vi "纳清DO电极校准.vi"() -> ()   [LabVIEW 2016, in "斯坦道多参数.lvlib"]
uses:
  <vilib>/Utility/miscctls.llb/LVPointTypeDef.ctl
  <vilib>/Utility/miscctls.llb/LVPositionTypeDef.ctl
  <vilib>/Analysis/NI_AALBase.lvlib
panel:
  out "盐度":sgl format="%#.2f"
  out "大气压力":sgl format="%#.2f"
  out "饱和值":sgl format="%#.2f"
  out "当前探头类别":string
  out "报警信息":string
  out "温度校准参数":sgl format="%#.2f"
  out "通讯状态":string
  out "第二点校准值":dbl
  out "第一点校准值":dbl
  in  "校准停止":bool
  in  "校准启动":bool
  in  "校准模式":enum16{"两点校准", "单点校准"}(ring)=enum."单点校准"
  out "最小值":sgl format="%#.2f"
  out "最大值":sgl format="%#.2f"
  out "波形图表":sgl(graph) caption="历史曲线"
  out "mean":dbl caption="均值" format="%#.2f"
  out "standard deviation":dbl caption="标准差" format="%#.2f"
  out "变异系数":dbl format="%#.6f"
  out "测量值":sgl format="%#.2f"
  out "提示":string
  out "原始光强数值":sgl caption="信号值" format="%#.6f"
  out "温度":dbl format="%#.2f"
  # "DO电极设定"
  # "℃"
  # "mg/L"
  # "%"
  # "nA"
  # "kPa"
  # "ppt"
  # "请选择校准模式:"
  # "℃"
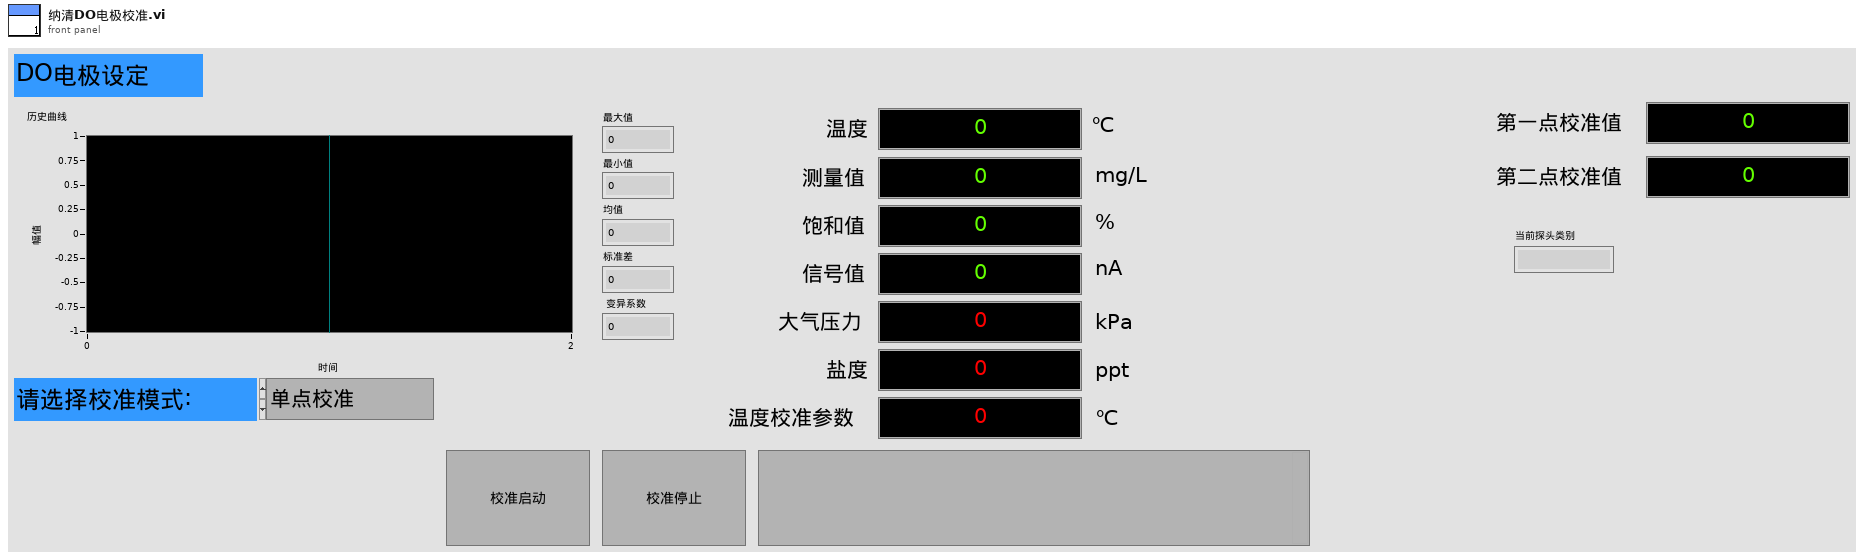
[diagram p1: front panel]
types:
  T1 = typedef "LVPointTypeDef.ctl" = cluster{"Horizontal":i16, "Vertical":i16}
  T2 = typedef "斯坦道多参数.lvlib/校准步骤.ctl" = enum16{"待机", "放置第一点标液", "第一点校准启动", "第一点校准写入", "第一点校准失败", "放置第二点标液", "第二点校准启动", "第二点校准写入", "第二点校准失败", "放置第三点标液", "第三点校准启动", "第三点校准写入", "第三点校准失败", "校准结果写入", "校准结束"}
  T3 = cluster{"报警码":u16, "溶解氧数值（mg/L）":sgl, "溶解氧数据（%）":sgl, "温度数据":sgl, "溶解氧原始信号 nA":sgl, "大气压力":sgl, "盐度":sgl, "0X0009_NC":string, "产品名称":string, "序列号":string, "硬件版本":string, "软件版本":string, "通讯地址":u16, "波特率":u16, "设备类型":u16, "0X0026_NC":string, "第一点原始数据":sgl, "第一点校准数据":sgl, "第二点原始数据":sgl, "第二点校准数据":sgl, "探头校准命令":u16, "温度校准参数":sgl, "温度校准命令":u16}
  T4 = typedef "LVPositionTypeDef.ctl" = cluster{"Left":i32, "Top":i32}
  T5 = cluster{"报警码":u16, "溶解氧数值（mg/L）":sgl, "溶解氧数据（%）":sgl, "温度数据":sgl, "溶解氧原始信号 nA":sgl, "大气压力":sgl, "盐度":sgl, "0X0009_NC":string, "产品名称":string, "序列号":string, "硬件版本":string, "软件版本":string, "通讯地址":u16, "波特率":u16, "设备类型":u16, "0X0026_NC":string, "第一点原始数据":sgl, "0X0033 NC":sgl, "第二点原始数据":sgl, "0X0037 NC":sgl, "探头校准命令":u16, "温度校准参数":sgl, "温度校准命令":u16}
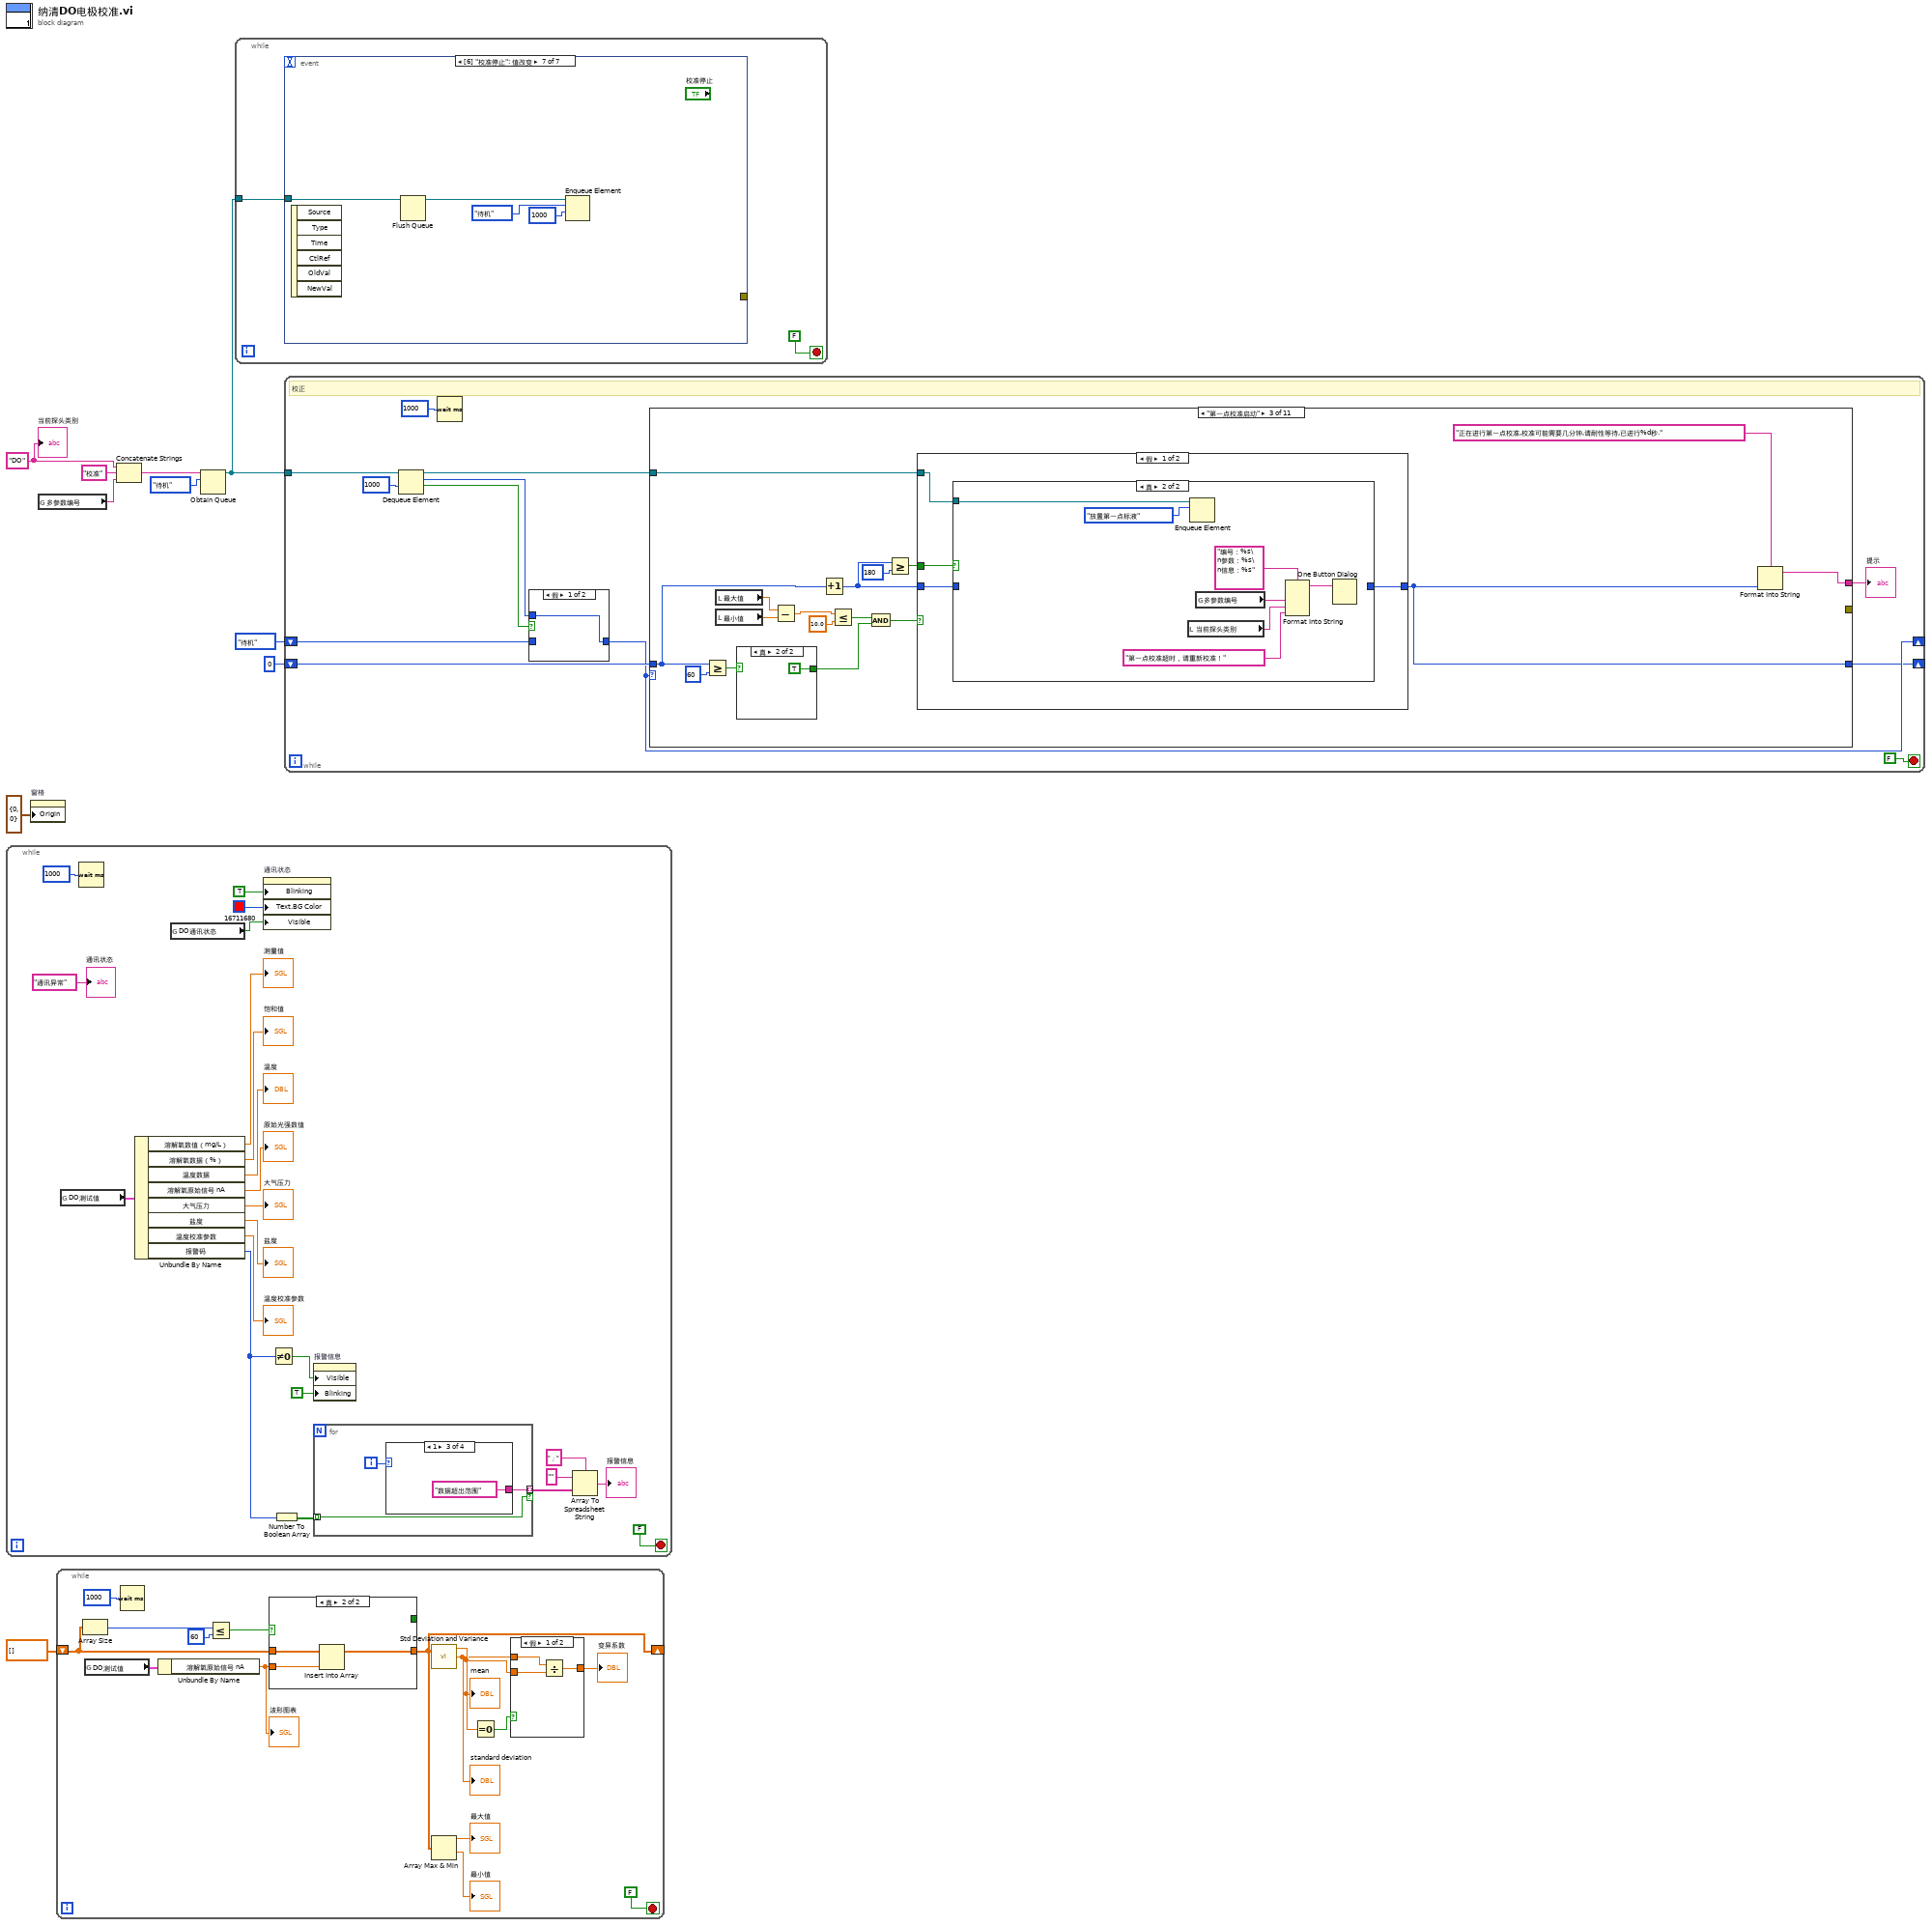
[diagram p0: block diagram]
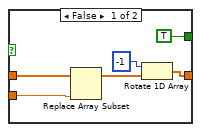
[diagram p3: hidden frame]
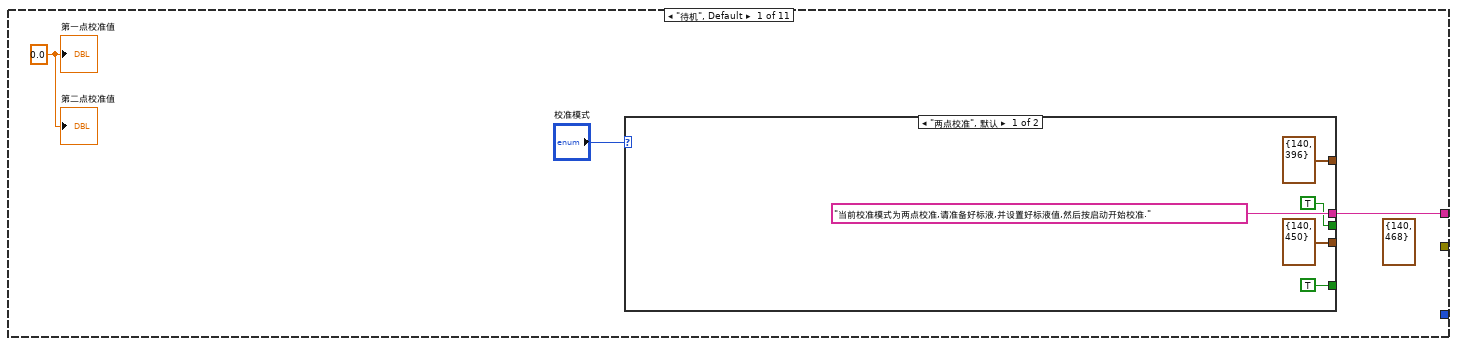
[diagram p5: hidden frame]
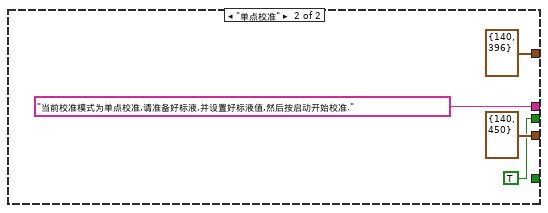
[diagram p6: hidden frame]
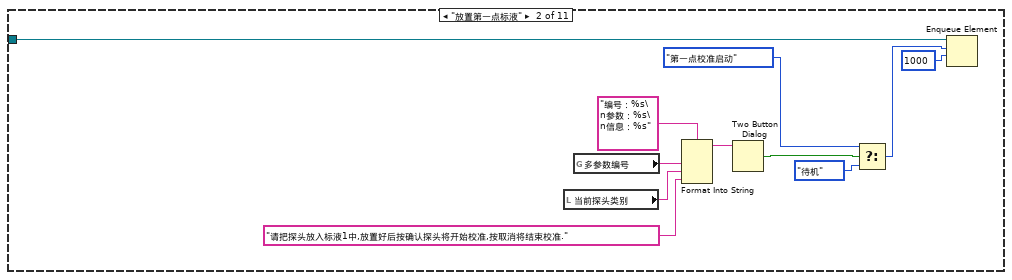
[diagram p7: hidden frame]
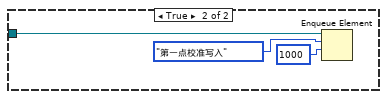
[diagram p9: hidden frame]
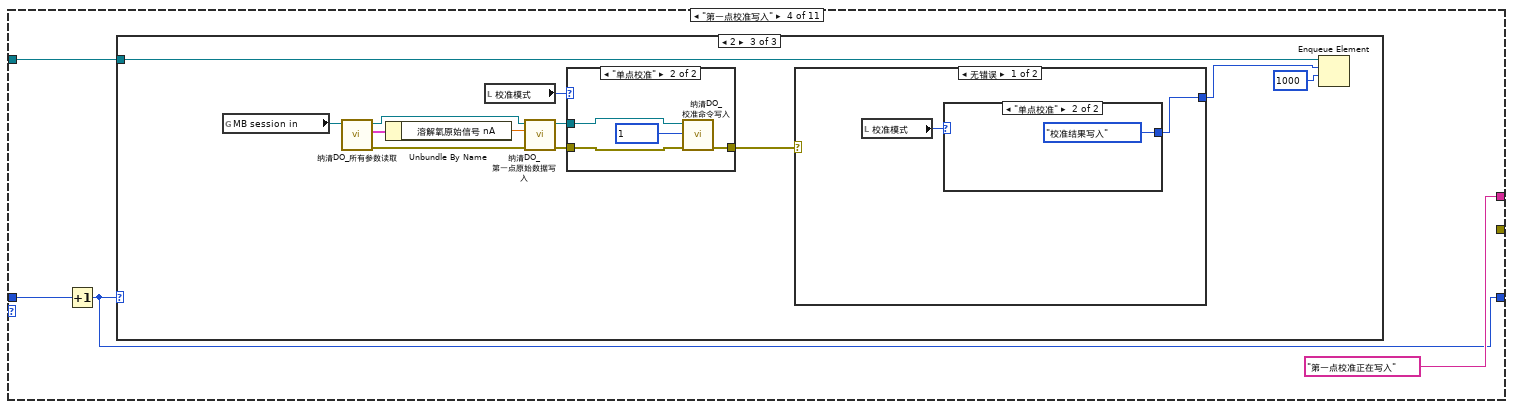
[diagram p11: hidden frame]
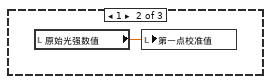
[diagram p13: hidden frame]
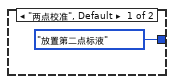
[diagram p15: hidden frame]
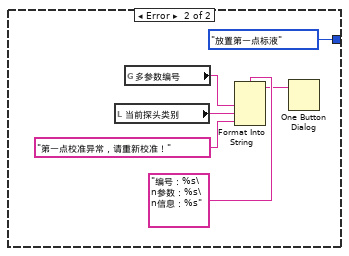
[diagram p16: hidden frame]
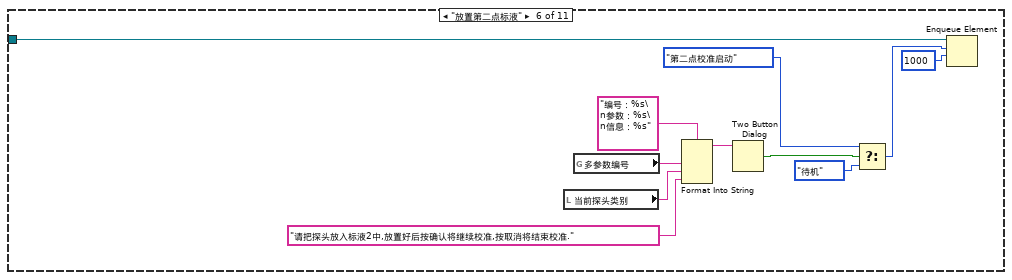
[diagram p18: hidden frame]
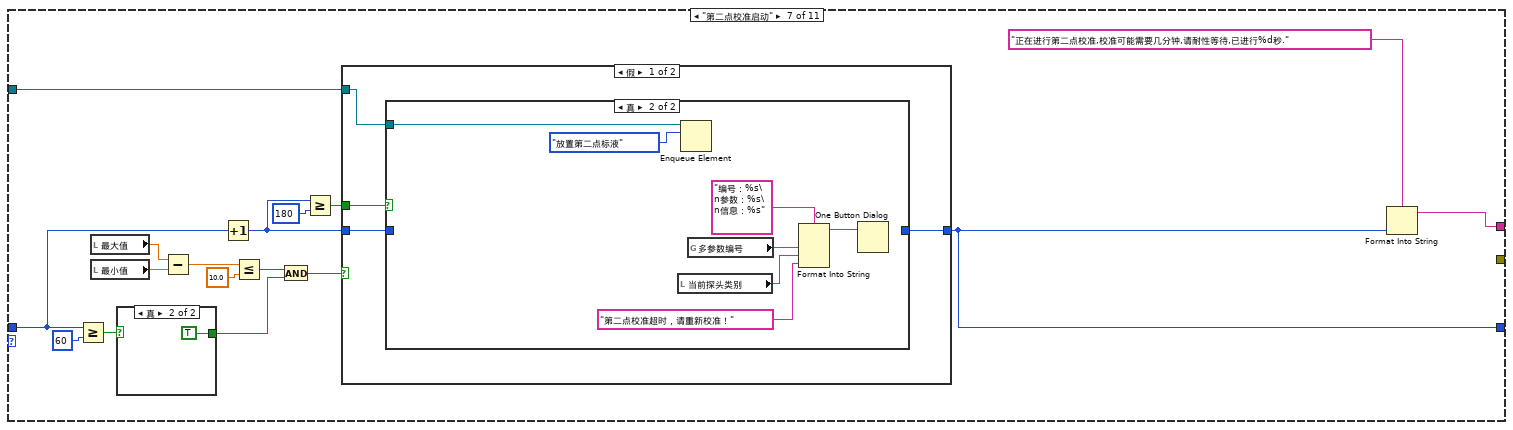
[diagram p19: hidden frame]
diagram:
  w1 = "DO" ("当前探头类别")
  n1 = while {
    stop <- FALSE stop-if-true
    n2 = global read "纳清过程全局变量.vi" "DO测试值"() -> (w30:T3)
    n3 = Wait (ms)(milliseconds to wait=u32 1000 ("等待时间（毫秒）")) -> ()  [unwired: 1 out]
    n4 = Unbundle By Name(w30) -> ("溶解氧数值（mg/L）"=→"测量值":sgl, "溶解氧数据（%）"=→"饱和值":sgl, "温度数据"=→"温度":sgl, "溶解氧原始信号 nA"=→"原始光强数值":sgl, "大气压力"=→"大气压力":sgl, "盐度"=→"盐度":sgl, "温度校准参数"=→"温度校准参数":sgl, "报警码"=w16:u16)
    n5 = global read "多参数全局变量.vi" "DO通讯状态"() -> (w23:bool)
    n6 = property on="通讯状态" class="Str"("Blinking"=TRUE ("闪烁"), "Text.BG Color"=u32 16711680, "Visible"=w23) -> ()  [unwired: 2 in, 2 out]
    n7 = Not Equal To 0?(x=w16) -> (x != 0?=w15:bool)
    n8 = Number To Boolean Array(number=w16) -> (Boolean array=w21:bool[])
    n9 = property on="报警信息" class="Str"("Visible"=w15, "Blinking"=TRUE ("闪烁")) -> ()  [unwired: 2 in, 2 out]
    n10 = for {
      tunnel: w21 -> [w33] mode=indexing
      tunnel: [w34] -> w20 mode=indexing if=w33
      i -> [w35]
      n11 = case shown="1" w35 {
        tunnel: [_ "温度超出范围" "数据超出范围" "温度传感器故障"] -> w34
        frame Default {
        }
        frame 0 {
        }
        frame 1 {
        }
        frame 8 {
        }
      }
    }
    n12 = Array To Spreadsheet String(delimiter (Tab)="；" ("分隔符(Tab)"), array=w20, 3:"" ("格式字符串")) -> (spreadsheet string=→"报警信息":string)
    "通讯状态" <- "通讯异常" ("当前串口")
  }
  n13 = property on="窗格" class="Pane"("Origin"=T1 {"Horizontal"=0, "Vertical"=0} ("原点")) -> ()  [unwired: 2 in, 2 out]
  n14 = global read "多参数全局变量.vi" "多参数编号"() -> (w2:string)
  n15 = while {
    shift-right: [w43] -> _
    shift-left: sgl[] [] -> [w49]
    stop <- FALSE stop-if-true
    n16 = Array Size(array=w49) -> (size(s)=w51:i32)
    n17 = global read "纳清过程全局变量.vi" "DO测试值"() -> (w39:T3)
    n18 = Wait (ms)(milliseconds to wait=u32 1000 ("等待时间（毫秒）")) -> ()  [unwired: 1 out]
    n19 = Unbundle By Name(w39) -> ("溶解氧原始信号 nA"=w40:sgl)
    "波形图表" <- w40
    n20 = Less Or Equal?(x=w51, y=60) -> (x <= y?=w50:bool)
    n21 = case shown="真" w50 {
      tunnel: w49 -> [w62 w65]
      tunnel: w40 -> [w60 w64]
      tunnel: [w58 w63] -> w43
      tunnel: [TRUE _] -> _
      frame False {
        n22 = Replace Array Subset(array=w62, new element=w60) -> (w61:sgl[])  [unwired: 1 in]
        n23 = Rotate 1D Array(1:w61, 2:-1 ("n")) -> (0:w58:sgl[])
      }
      frame True {
        n24 = Insert Into Array(array=w65, new element=w64) -> (w63:sgl[])  [unwired: 1 in]
      }
    }
    n25 = call <vilib>:"Std Deviation and Variance.vi"("X"=w43) -> ("mean"=w47:dbl, "standard deviation"=w46:dbl)  [unwired: 1 in, 1 out]
    "mean" <- w47
    "standard deviation" <- w46
    n26 = Array Max & Min(array=w43) -> (max value=→"最大值":sgl, min value=→"最小值":sgl)  [unwired: 2 out]
    n27 = Equal To 0?(x=w47) -> (x = 0?=w48:bool)
    n28 = case shown="假" w48 {
      tunnel: w46 -> [w56 _]
      tunnel: [w55 _] -> w45
      tunnel: w47 -> [w54 _]
      frame False {
        n29 = Divide(x=w56, y=w54) -> (x/y=w55:dbl)
      }
      frame True {
      }
    }
    "变异系数" <- w45
  }
  n30 = Concatenate Strings(w1, "校准" ("名称（未命名）"), w2) -> (w3:string)
  n31 = Obtain Queue(name (unnamed)=w3, element data type=校准步骤."待机" ("枚举")) -> (queue out=w5:refnum<queue>)  [unwired: 3 in, 2 out]
  n32 = while {
    tunnel: w5 -> [w66]
    stop <- FALSE stop-if-true
    n33 = event shown="[6] \"校准停止\": 值改变" {
      selector: _ -> [_ _ _ _ _ _ _]
      dyn-events: _ -> [_ _ _ _ _ _ _]
      timeout: _ -> [_ _ _ _ _ _ _]
      tunnel: [_ _ w73 w77 w78 _ _] -> _
      tunnel: w66 -> [_ _ _ _ _ w85 w87]
      event Timeout {
        n34 = event-data() -> ()  [unwired: 1 in, 3 out]
      }
      event "温度校准参数", "大气压力", "饱和值": Mouse Down {
        n35 = event-data() -> ("CtlRef"=w68:refnum<vi>)  [unwired: 1 in, 7 out]
        n36 = property class="DigNum (严格)"(reference=w68) -> (reference out=w69:refnum<vi>, "Value"=w70:sgl)  [unwired: 1 in, 1 out]
        n37 = call "数字键盘.vi"("OldNumber"=w70) -> ("NewNumber"=w71:dbl)  [unwired: 1 in]
        n38 = property class="DigNum (严格)"(reference=w69, "Val(Sgnl)"=w71) -> ()  [unwired: 1 in, 2 out]
      }
      event "大气压力": Value Change {
        n39 = event-data() -> ("NewVal"=w72:sgl)  [unwired: 1 in, 5 out]
        n40 = global read "多参数全局变量.vi" "MB session in"() -> (w74:refnum<class "MB_Master.lvclass">)
        n41 = call "纳清DO_大气压力写入.vi"("数值"=w72, "MB session in"=w74) -> ("error out"=w73:errorcluster)  [unwired: 8 in, 1 out]
      }
      event "盐度": Value Change {
        n42 = event-data() -> ("NewVal"=w75:sgl)  [unwired: 1 in, 5 out]
        n43 = global read "多参数全局变量.vi" "MB session in"() -> (w76:refnum<class "MB_Master.lvclass">)
        n44 = call "纳清DO_盐度写入.vi"("数值"=w75, "MB session in"=w76) -> ("error out"=w77:errorcluster)  [unwired: 8 in, 1 out]
      }
      event "温度校准参数": Value Change {
        n45 = event-data() -> ("NewVal"=w83:sgl)  [unwired: 1 in, 5 out]
        n46 = global read "多参数全局变量.vi" "MB session in"() -> (w82:refnum<class "MB_Master.lvclass">)
        n47 = call "纳清DO_温度校准参数写入.vi"("数值"=w83, "MB session in"=w82) -> ("error out"=w84:errorcluster, "MB session out"=w81:refnum<class "MB_Master.lvclass">)  [unwired: 8 in]
        n48 = call "纳清DO_温度校准命令写入.vi"("error in (no error)"=w84, "数值"=u16 1 ("starting address"), "MB session in"=w81) -> ("error out"=w79:errorcluster)  [unwired: 7 in, 1 out]
        n49 = call <vilib>:"Simple Error Handler.vi"("error in (no error)"=w79) -> ("error out"=w78:errorcluster)  [unwired: 4 in, 4 out]
      }
      event "校准启动": Value Change {
        n50 = event-data() -> ()  [unwired: 1 in, 6 out]
        n51 = Enqueue Element(queue=w85, element=校准步骤."放置第一点标液" ("元素")) -> ()  [unwired: 2 in, 3 out]
      }
      event "校准停止": Value Change {
        n52 = event-data() -> ()  [unwired: 1 in, 6 out]
        n53 = Flush Queue(queue=w87) -> (queue out=w88:refnum<queue>)  [unwired: 1 in, 2 out]
        n54 = Enqueue Element(queue=w88, element=校准步骤."待机" ("元素"), timeout in ms (-1)=1000 ("超时毫秒(-1)")) -> ()  [unwired: 1 in, 3 out]
      }
    }
  }
  n55 = while "While循环" {
    shift-right: [w92] -> _
    shift-left: 校准步骤."待机" ("枚举") -> [w94]
    shift-right: [w91] -> _
    shift-left: 0 -> [w100]
    tunnel: w5 -> [w95]
    stop <- FALSE stop-if-true
    # "校正"
    n56 = Dequeue Element(queue=w95, timeout in ms (-1)=1000 ("超时毫秒(-1)")) -> (queue out=w93:refnum<queue>, element=w96:T2, timed out?=w97:bool)  [unwired: 1 in, 1 out]
    n57 = Wait (ms)(milliseconds to wait=u32 1000 ("等待时间（毫秒）")) -> ()  [unwired: 1 out]
    n58 = case shown="假" w97 {
      tunnel: w96 -> [w103 _]
      tunnel: [w103 w104] -> w92
      tunnel: w94 -> [_ w104]
      frame False {
      }
      frame True {
      }
    }
    n59 = case shown="\"第一点校准启动\"" w92 {
      tunnel: [w106 _ w129 "第一点校准正在写入" ("提示") _ _ w206 "第二点校准正在写入" ("提示") "第二点校准失败" ("提示") w272 w287] -> w99
      tunnel: w100 -> [_ _ w130 w163 _ _ w207 w239 _ _ _]
      tunnel: [_ _ w128 w161 _ _ w205 w237 _ _ _] -> w91
      tunnel: w93 -> [_ w123 w131 w162 _ w198 w208 w238 _ w278 _]
      tunnel: [_ _ _ _ _ _ _ _ _ w276 _] -> _
      frame "待机", Default {
        (unwired) T4 {"Left"=140, "Top"=468} ("位置 3")
        w105 = 0.0 ("第一点校准值")
        n60 = case shown="\"两点校准\", 默认" "校准模式" {
          tunnel: ["当前校准模式为两点校准,请准备好标液,并设置好标液值,然后按启动开始校准." ("提示") "当前校准模式为单点校准,请准备好标液,并设置好标液值,然后按启动开始校准." ("提示")] -> w106
          tunnel: [TRUE ("可见") _] -> _
          tunnel: [T4 {"Left"=140, "Top"=396} ("位置") T4 {"Left"=140, "Top"=396} ("位置")] -> _
          tunnel: [T4 {"Left"=140, "Top"=450} ("位置 2") T4 {"Left"=140, "Top"=450} ("位置 2")] -> _
          tunnel: [TRUE ("可见") TRUE ("可见")] -> _
          frame "两点校准", Default {
          }
          frame "单点校准" {
          }
        }
        "第一点校准值" <- w105
        "第二点校准值" <- w105
      }
      frame "放置第一点标液" {
        n61 = local read "当前探头类别"() -> (w117:string)
        n62 = global read "多参数全局变量.vi" "多参数编号"() -> (w121:string)
        n63 = Format Into String(format string="编号：%s\n参数：%s\n信息：%s" ("格式字符串"), w121, w117, "请把探头放入标液1中,放置好后按确认探头将开始校准,按取消将结束校准." ("消息")) -> (resulting string=w120:string)  [unwired: 2 in, 1 out]
        n64 = Two Button Dialog(message=w120) -> (T button?=w118:bool)  [unwired: 2 in]
        n65 = Select(t=校准步骤."第一点校准启动" ("元素"), s=w118, f=校准步骤."待机" ("元素")) -> (s? t:f=w124:T2)
        n66 = Enqueue Element(queue=w123, element=w124, timeout in ms (-1)=1000 ("超时毫秒(-1)")) -> ()  [unwired: 1 in, 3 out]
      }
      frame "第一点校准启动" {
        n67 = Greater Or Equal?(x=w130, y=60) -> (x >= y?=w137:bool)
        n68 = local read "最大值"() -> (w140:sgl)
        n69 = local read "最小值"() -> (w139:sgl)
        n70 = case shown="真" w137 {
          tunnel: [_ TRUE] -> w138
          frame False {
          }
          frame True {
          }
        }
        n71 = Subtract(x=w140, y=w139) -> (x-y=w141:sgl)
        n72 = Increment(x=w130) -> (x+1=w144:i32)
        n73 = Less Or Equal?(x=w141, y=10.0) -> (x <= y?=w134:bool)
        n74 = And(x=w134, y=w138) -> (x .and. y?=w142:bool)
        n75 = Greater Or Equal?(x=w144, y=180) -> (x >= y?=w143:bool)
        n76 = case shown="假" w142 {
          tunnel: w131 -> [w147 w159]
          tunnel: w143 -> [w148 _]
          tunnel: w144 -> [w146 _]
          tunnel: [w145 _] -> w128
          frame False {
            n77 = case shown="真" w148 {
              tunnel: w147 -> [_ w156]
              tunnel: w146 -> [w149 _]
              tunnel: [w149 _] -> w145
              frame False {
              }
              frame True {
                n78 = local read "当前探头类别"() -> (w150:string)
                n79 = Enqueue Element(queue=w156, element=校准步骤."放置第一点标液" ("元素")) -> ()  [unwired: 2 in, 3 out]
                n80 = global read "多参数全局变量.vi" "多参数编号"() -> (w153:string)
                n81 = Format Into String(format string="编号：%s\n参数：%s\n信息：%s" ("格式字符串"), w153, w150, "第一点校准超时，请重新校准！" ("error source (\" \")")) -> (resulting string=w151:string)  [unwired: 2 in, 1 out]
                n82 = One Button Dialog(message=w151) -> ()  [unwired: 1 in, 1 out]
              }
            }
          }
          frame True {
            n83 = Enqueue Element(queue=w159, element=校准步骤."第一点校准写入" ("元素"), timeout in ms (-1)=1000 ("超时毫秒(-1)")) -> ()  [unwired: 1 in, 3 out]
          }
        }
        n84 = Format Into String(format string="正在进行第一点校准,校准可能需要几分钟,请耐性等待,已进行%d秒." ("格式字符串"), w128) -> (resulting string=w129:string)  [unwired: 2 in, 1 out]
      }
      frame "第一点校准写入" {
        n85 = Increment(x=w163) -> (x+1=w161:i32)
        n86 = case shown="2" w161 {
          tunnel: w162 -> [_ _ w177]
          frame 0, Default {
          }
          frame 1 {
            n87 = local read "原始光强数值"() -> (w165:sgl)
            n88 = local write "第一点校准值"(w165) -> ()
          }
          frame 2 {
            n89 = global read "多参数全局变量.vi" "MB session in"() -> (w173:refnum<class "MB_Master.lvclass">)
            n90 = call "纳清DO_所有参数读取.vi"("MB session in"=w173) -> ("error out"=w175:errorcluster, "输出值"=w172:T5, "MB session out"=w174:refnum<class "MB_Master.lvclass">)  [unwired: 8 in]
            n91 = Unbundle By Name(w172) -> ("溶解氧原始信号 nA"=w171:sgl)
            n92 = local read "校准模式"() -> (w166:enum16{"两点校准", "单点校准"})
            n93 = call "纳清DO_第一点原始数据写入.vi"("error in (no error)"=w175, "数值"=w171, "MB session in"=w174) -> ("error out"=w170:errorcluster, "MB session out"=w169:refnum<class "MB_Master.lvclass">)  [unwired: 7 in]
            n94 = case shown="\"单点校准\"" w166 {
              tunnel: w170 -> [w178 w182]
              tunnel: w169 -> [_ w181]
              tunnel: [w178 w179] -> w168
              frame "两点校准", Default {
              }
              frame "单点校准" {
                n95 = call "纳清DO_校准命令写入.vi"("error in (no error)"=w182, "数值"=u16 1 ("starting address"), "MB session in"=w181) -> ("error out"=w179:errorcluster)  [unwired: 7 in, 1 out]
              }
            }
            n96 = case shown="无错误" w168 {
              tunnel: [w183 校准步骤."放置第一点标液" ("元素")] -> w167
              frame No Error {
                n97 = local read "校准模式"() -> (w184:enum16{"两点校准", "单点校准"})
                n98 = case shown="\"单点校准\"" w184 {
                  tunnel: [校准步骤."放置第二点标液" ("元素") 校准步骤."校准结果写入" ("元素")] -> w183
                  frame "两点校准", Default {
                  }
                  frame "单点校准" {
                  }
                }
              }
              frame Error {
                n99 = local read "当前探头类别"() -> (w187:string)
                n100 = global read "多参数全局变量.vi" "多参数编号"() -> (w191:string)
                n101 = Format Into String(format string="编号：%s\n参数：%s\n信息：%s" ("格式字符串"), w191, w187, "第一点校准异常，请重新校准！" ("error source (\" \")")) -> (resulting string=w189:string)  [unwired: 2 in, 1 out]
                n102 = One Button Dialog(message=w189) -> ()  [unwired: 1 in, 1 out]
              }
            }
            n103 = Enqueue Element(queue=w177, element=w167, timeout in ms (-1)=1000 ("超时毫秒(-1)")) -> ()  [unwired: 1 in, 3 out]
          }
        }
      }
      frame "第一点校准失败" {
      }
      frame "放置第二点标液" {
        n104 = local read "当前探头类别"() -> (w193:string)
        n105 = global read "多参数全局变量.vi" "多参数编号"() -> (w196:string)
        n106 = Format Into String(format string="编号：%s\n参数：%s\n信息：%s" ("格式字符串"), w196, w193, "请把探头放入标液2中,放置好后按确认将继续校准,按取消将结束校准." ("消息")) -> (resulting string=w195:string)  [unwired: 2 in, 1 out]
        n107 = Two Button Dialog(message=w195) -> (T button?=w202:bool)  [unwired: 2 in]
        n108 = Select(t=校准步骤."第二点校准启动" ("元素"), s=w202, f=校准步骤."待机" ("元素")) -> (s? t:f=w199:T2)
        n109 = Enqueue Element(queue=w198, element=w199, timeout in ms (-1)=1000 ("超时毫秒(-1)")) -> ()  [unwired: 1 in, 3 out]
      }
      frame "第二点校准启动" {
        n110 = Greater Or Equal?(x=w207, y=60) -> (x >= y?=w213:bool)
        n111 = local read "最大值"() -> (w216:sgl)
        n112 = local read "最小值"() -> (w215:sgl)
        n113 = case shown="真" w213 {
          tunnel: [_ TRUE] -> w214
          frame False {
          }
          frame True {
          }
        }
        n114 = Subtract(x=w216, y=w215) -> (x-y=w217:sgl)
        n115 = Increment(x=w207) -> (x+1=w220:i32)
        n116 = Less Or Equal?(x=w217, y=10.0) -> (x <= y?=w210:bool)
        n117 = And(x=w210, y=w214) -> (x .and. y?=w218:bool)
        n118 = Greater Or Equal?(x=w220, y=180) -> (x >= y?=w219:bool)
        n119 = case shown="假" w218 {
          tunnel: w208 -> [w223 w235]
          tunnel: w219 -> [w224 _]
          tunnel: w220 -> [w222 _]
          tunnel: [w221 _] -> w205
          frame False {
            n120 = case shown="真" w224 {
              tunnel: w223 -> [_ w232]
              tunnel: w222 -> [w225 _]
              tunnel: [w225 _] -> w221
              frame False {
              }
              frame True {
                n121 = local read "当前探头类别"() -> (w226:string)
                n122 = Enqueue Element(queue=w232, element=校准步骤."放置第二点标液" ("元素")) -> ()  [unwired: 2 in, 3 out]
                n123 = global read "多参数全局变量.vi" "多参数编号"() -> (w229:string)
                n124 = Format Into String(format string="编号：%s\n参数：%s\n信息：%s" ("格式字符串"), w229, w226, "第二点校准超时，请重新校准！" ("消息")) -> (resulting string=w228:string)  [unwired: 2 in, 1 out]
                n125 = One Button Dialog(message=w228) -> ()  [unwired: 1 in, 1 out]
              }
            }
          }
          frame True {
            n126 = Enqueue Element(queue=w235, element=校准步骤."第二点校准写入" ("元素"), timeout in ms (-1)=1000 ("超时毫秒(-1)")) -> ()  [unwired: 1 in, 3 out]
          }
        }
        n127 = Format Into String(format string="正在进行第二点校准,校准可能需要几分钟,请耐性等待,已进行%d秒." ("格式字符串"), w205) -> (resulting string=w206:string)  [unwired: 2 in, 1 out]
      }
      frame "第二点校准写入" {
        n128 = Increment(x=w239) -> (x+1=w237:i32)
        n129 = case shown="2" w237 {
          tunnel: w238 -> [_ _ w253]
          frame 0, Default {
          }
          frame 1 {
            n130 = local read "原始光强数值"() -> (w241:sgl)
            n131 = local write "第二点校准值"(w241) -> ()
          }
          frame 2 {
            n132 = global read "多参数全局变量.vi" "MB session in"() -> (w249:refnum<class "MB_Master.lvclass">)
            n133 = call "纳清DO_所有参数读取.vi"("MB session in"=w249) -> ("error out"=w251:errorcluster, "输出值"=w248:T5, "MB session out"=w250:refnum<class "MB_Master.lvclass">)  [unwired: 8 in]
            n134 = Unbundle By Name(w248) -> ("溶解氧原始信号 nA"=w247:sgl)
            n135 = local read "校准模式"() -> (w242:enum16{"两点校准", "单点校准"})
            n136 = call "纳清DO_第二点原始数据写入.vi"("error in (no error)"=w251, "数值"=w247, "MB session in"=w250) -> ("error out"=w246:errorcluster, "MB session out"=w245:refnum<class "MB_Master.lvclass">)  [unwired: 7 in]
            n137 = case shown="\"两点校准\"" w242 {
              tunnel: w246 -> [w257 w258]
              tunnel: w245 -> [w256 _]
              tunnel: [w254 w258] -> w244
              frame "两点校准" {
                n138 = call "纳清DO_校准命令写入.vi"("error in (no error)"=w257, "数值"=u16 2 ("starting address"), "MB session in"=w256) -> ("error out"=w254:errorcluster)  [unwired: 7 in, 1 out]
              }
              frame "单点校准", Default {
              }
            }
            n139 = case shown="错误" w244 {
              tunnel: [w259 校准步骤."放置第二点标液" ("元素")] -> w243
              frame No Error {
                n140 = local read "校准模式"() -> (w260:enum16{"两点校准", "单点校准"})
                n141 = case shown="\"单点校准\"" w260 {
                  tunnel: [校准步骤."校准结果写入" ("元素") 校准步骤."校准结果写入" ("元素")] -> w259
                  frame "两点校准", Default {
                  }
                  frame "单点校准" {
                  }
                }
              }
              frame Error {
                n142 = local read "当前探头类别"() -> (w263:string)
                n143 = global read "多参数全局变量.vi" "多参数编号"() -> (w267:string)
                n144 = Format Into String(format string="编号：%s\n参数：%s\n信息：%s" ("格式字符串"), w267, w263, "第二点校准异常，请重新校准！" ("error source (\" \")")) -> (resulting string=w265:string)  [unwired: 2 in, 1 out]
                n145 = One Button Dialog(message=w265) -> ()  [unwired: 1 in, 1 out]
              }
            }
            n146 = Enqueue Element(queue=w253, element=w243, timeout in ms (-1)=1000 ("超时毫秒(-1)")) -> ()  [unwired: 1 in, 3 out]
          }
        }
      }
      frame "第二点校准失败" {
      }
      frame "校准结果写入" {
        n147 = Enqueue Element(queue=w278, element=校准步骤."校准结束" ("元素")) -> ()  [unwired: 2 in, 3 out]
        n148 = local read "校准模式"() -> (w277:enum16{"两点校准", "单点校准"})
        n149 = case shown="\"两点校准\", 默认" w277 {
          tunnel: [w281 w286] -> w273
          frame "两点校准", Default {
            n150 = local read "第一点校准值"() -> (w283:dbl)
            n151 = local read "第二点校准值"() -> (w280:dbl)
            n152 = Format Into String(format string="校准结果：第一点校准值=%f，第一点标准值=0%%,第二点校准值=%f，第二点标准值=100%%." ("提示"), w283, w280) -> (resulting string=w281:string)  [unwired: 2 in, 1 out]
          }
          frame "单点校准" {
            n153 = local read "第一点校准值"() -> (w285:dbl)
            n154 = Format Into String(format string="校准结果：校准值=%f，标准值=100%%。" ("提示"), w285) -> (resulting string=w286:string)  [unwired: 2 in, 1 out]
          }
        }
        n155 = local read "当前探头类别"() -> (w270:string)
        n156 = global read "多参数全局变量.vi" "多参数编号"() -> (w274:string)
        n157 = Format Into String(format string="编号：%s\n参数：%s\n信息：%s" ("格式字符串"), w274, w270, w273) -> (resulting string=w272:string)  [unwired: 2 in, 1 out]
        n158 = One Button Dialog(message=w272) -> ()  [unwired: 1 in, 1 out]
        n159 = call "操作日志.vi"("table"="校准记录", "日志信息"=w272) -> ("error out"=w276:errorcluster)  [unwired: 9 in]
      }
      frame "校准结束" {
        n160 = local read "提示"() -> (w287:string)
      }
    }
    "提示" <- w99
  }
  "当前探头类别" <- w1
